vi "Unpack Actor Data Msg.vi"(11 "Actor Data Msg":refnum<class "Observe Data Msg.lvclass">) -> (1 "Publication Time":timestamp, 2 "Value":variant, 3 "Datum Name":string)   [LabVIEW 2017, in "IObserver.lvlib" / "Observe Data Msg.lvclass"]
doc: "<License>\nCopyright © 2017 Composed Systems, LLC | All rights reserved\nwww.composed.io\n\nAuthor: Ethan Stern <ethan.stern@composed.io>\n\nThis software is provided \"AS IS\" WITHOUT WARRANTIES, either express or implied, AND IS FOR EDUCATIONAL PURPOSES ONLY.\n</License>"
uses:
  Observe Data Msg.lvclass
  Observe Data Msg.lvclass/Observe Data Msg.ctl
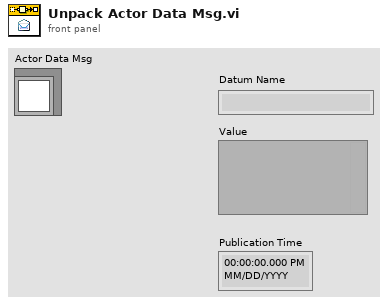
[diagram p1: front panel]
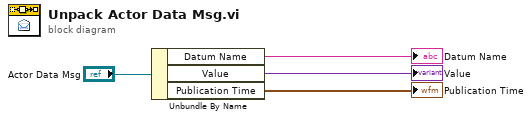
[diagram p0: block diagram]
diagram:
  n1 = Unbundle By Name("Actor Data Msg") -> ("Datum Name"=→"Datum Name":string, "Value"=→"Value":variant, "Publication Time"=→"Publication Time":timestamp)
